vi "Tiempos_Muertos.vi"(0 "Tiempos Muertos":T1={"T.M.CH1"=20, "T.M.CH2"=20, "T.M.CH3"=20, "T.M.CH4"=20, "T.M.CH5"=20, "T.M.CH6"=20, "T.M.CH7"=20, "T.M.CH8"=20} {"T.M.CH8" min=10 max=90 step=1; "T.M.CH7" min=10 max=90 step=1; "T.M.CH6" min=10 max=90 step=1; "T.M.CH5" min=10 max=90 step=1; "T.M.CH4" min=10 max=90 step=1; "T.M.CH3" min=10 max=90 step=1; "T.M.CH2" min=10 max=90 step=1; "T.M.CH1" min=10 max=90 step=1}, 1 "Min/Seg":u16, 5 "Error In":errorcluster) -> (19 "Error Out":errorcluster)   [LabVIEW 2013]
uses:
  Controles/Tiempos_Muertos_TB.ctl
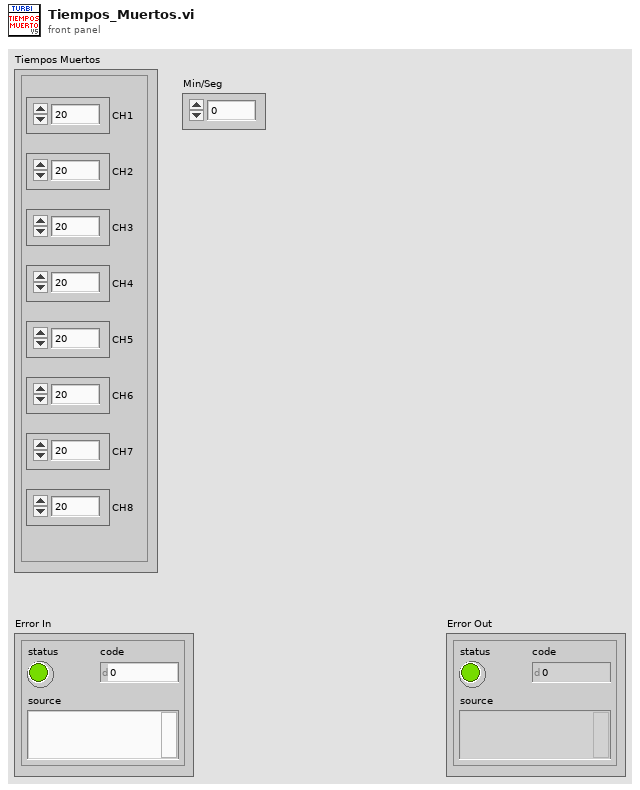
[diagram p1: front panel]
types:
  T1 = typedef "Tiempos_Muertos_TB.ctl" = cluster{"T.M.CH1":u8, "T.M.CH2":u8, "T.M.CH3":u8, "T.M.CH4":u8, "T.M.CH5":u8, "T.M.CH6":u8, "T.M.CH7":u8, "T.M.CH8":u8}
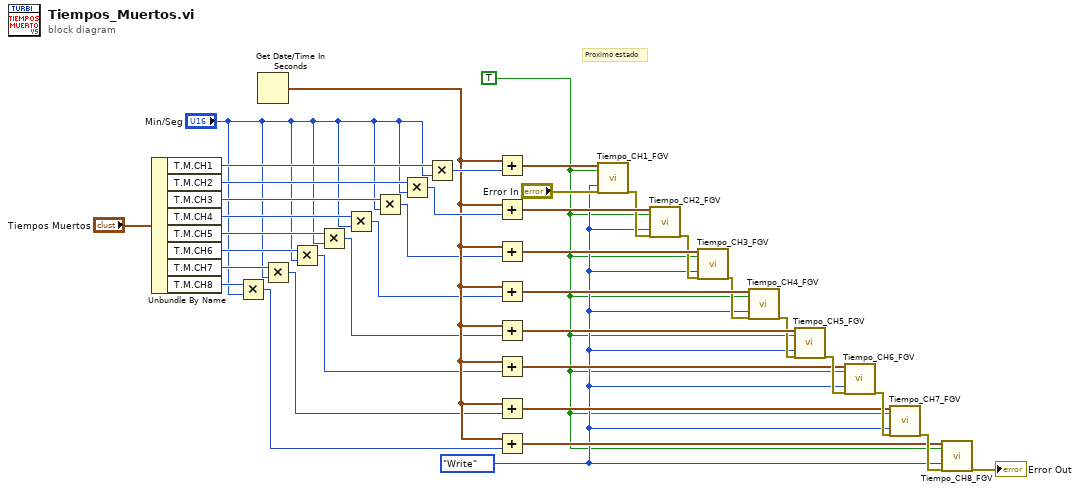
[diagram p0: block diagram]
diagram:
  w1 = TRUE ("Prox. Estado_IN")
  w2 = enum16{"Write", "Read"}."Write" ("Opción")
  # "Proximo estado"
  n1 = Unbundle By Name("Tiempos Muertos") -> ("T.M.CH1"=w37:u8, "T.M.CH2"=w34:u8, "T.M.CH3"=w31:u8, "T.M.CH4"=w30:u8, "T.M.CH5"=w29:u8, "T.M.CH6"=w28:u8, "T.M.CH7"=w27:u8, "T.M.CH8"=w26:u8)
  n2 = Multiply(x=w26, y="Min/Seg") -> (x*y=w19:u16)
  n3 = Get Date/Time In Seconds() -> (seconds since 1Jan1904=w32:timestamp)
  n4 = Multiply(x=w27, y="Min/Seg") -> (x*y=w20:u16)
  n5 = Multiply(x=w28, y="Min/Seg") -> (x*y=w21:u16)
  n6 = Multiply(x=w29, y="Min/Seg") -> (x*y=w22:u16)
  n7 = Multiply(x=w30, y="Min/Seg") -> (x*y=w23:u16)
  n8 = Multiply(x=w31, y="Min/Seg") -> (x*y=w24:u16)
  n9 = Multiply(x=w34, y="Min/Seg") -> (x*y=w33:u16)
  n10 = Multiply(x=w37, y="Min/Seg") -> (x*y=w36:u16)
  n11 = Add(x=w32, y=w36) -> (x+y=w35:timestamp)
  n12 = Add(x=w32, y=w33) -> (x+y=w18:timestamp)
  n13 = Add(x=w32, y=w24) -> (x+y=w16:timestamp)
  n14 = Add(x=w32, y=w23) -> (x+y=w13:timestamp)
  n15 = Add(x=w32, y=w22) -> (x+y=w11:timestamp)
  n16 = Add(x=w32, y=w21) -> (x+y=w8:timestamp)
  n17 = Add(x=w32, y=w20) -> (x+y=w6:timestamp)
  n18 = Add(x=w32, y=w19) -> (x+y=w3:timestamp)
  n19 = call "Tiempo_CH1_FGV.vi"("Tiempo_IN"=w35, "Prox. Estado_IN"=w1, "Opción"=w2, "Error In"="Error In") -> ("Error Out"=w15:errorcluster)  [unwired: 13 in, 2 out]
  n20 = call "Tiempo_CH2_FGV.vi"("Tiempo_IN"=w18, "Prox. Estado_IN"=w1, "Opción"=w2, "Error In"=w15) -> ("Error Out"=w14:errorcluster)  [unwired: 13 in, 2 out]
  n21 = call "Tiempo_CH3_FGV.vi"("Tiempo_IN"=w16, "Prox. Estado_IN"=w1, "Opción"=w2, "Error In"=w14) -> ("Error Out"=w12:errorcluster)  [unwired: 13 in, 2 out]
  n22 = call "Tiempo_CH4_FGV.vi"("Tiempo_IN"=w13, "Prox. Estado_IN"=w1, "Opción"=w2, "Error In"=w12) -> ("Error Out"=w10:errorcluster)  [unwired: 13 in, 2 out]
  n23 = call "Tiempo_CH5_FGV.vi"("Tiempo_IN"=w11, "Prox. Estado_IN"=w1, "Opción"=w2, "Error In"=w10) -> ("Error Out"=w9:errorcluster)  [unwired: 13 in, 2 out]
  n24 = call "Tiempo_CH6_FGV.vi"("Tiempo_IN"=w8, "Prox. Estado_IN"=w1, "Opción"=w2, "Error In"=w9) -> ("Error Out"=w7:errorcluster)  [unwired: 13 in, 2 out]
  n25 = call "Tiempo_CH7_FGV.vi"("Tiempo_IN"=w6, "Prox. Estado_IN"=w1, "Opción"=w2, "Error In"=w7) -> ("Error Out"=w5:errorcluster)  [unwired: 13 in, 2 out]
  n26 = call "Tiempo_CH8_FGV.vi"("Tiempo_IN"=w3, "Prox. Estado_IN"=w1, "Opción"=w2, "Error In"=w5) -> ("Error Out"=→"Error Out":errorcluster)  [unwired: 13 in, 2 out]
